vi "Input.vi"(8 "error in (no error)":errorcluster caption="错误输入（无错误）", 11 "Data In":T1) -> (0 "error out":errorcluster caption="错误输出", 3 "Data Out":T1)   [LabVIEW 2013]
uses:
  Control/Data.ctl
  Control/YV.ctl
  Control/SW.ctl
  Control/State.ctl
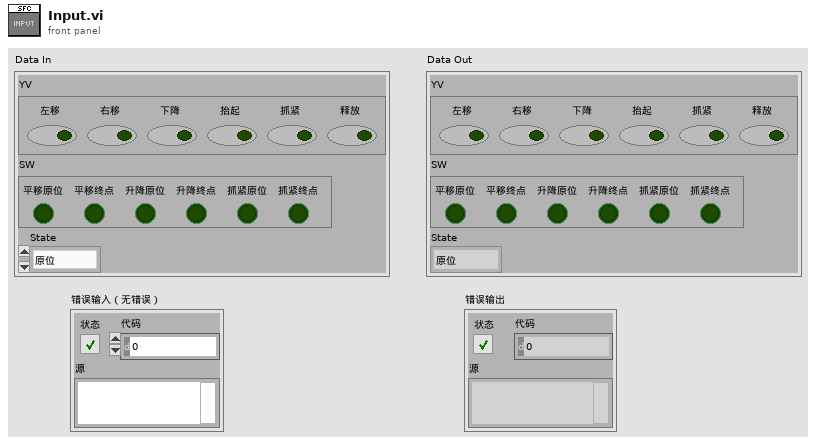
[diagram p1: front panel]
types:
  T1 = typedef "Data.ctl" = cluster{"YV":T2, "SW":T3, "State":T4}
  T2 = typedef "YV.ctl" = cluster{"左移":bool, "右移":bool, "下降":bool, "抬起":bool, "抓紧":bool, "释放":bool}
  T3 = typedef "SW.ctl" = cluster{"平移原位":bool, "平移终点":bool, "升降原位":bool, "升降终点":bool, "抓紧原位":bool, "抓紧终点":bool}
  T4 = typedef "State.ctl" = enum16{"原位", "A侧下降", "夹紧工件", "A侧抬起", "右移", "B侧下降", "释放工件", "B侧抬起", "左移"}
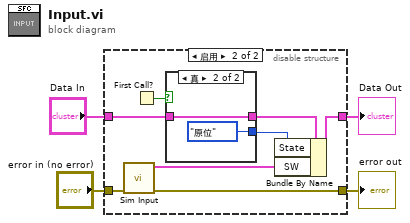
[diagram p0: block diagram]
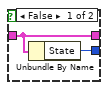
[diagram p3: hidden frame]
diagram:
  n1 = disable-structure shown="启用" {
    disable-tunnel: "Data In" -> [w6 w9]
    disable-tunnel: [w6 w14] -> w3
    disable-tunnel: "error in (no error)" -> [w5 w13]
    disable-tunnel: [w5 w12] -> w1
    frame Disabled {
    }
    frame Enabled {
      n2 = call "Sim Input.vi"("error in (no error)"=w13) -> ("error out"=w12:errorcluster, "SW Out"=w7:T3)  [unwired: 8 in]
      n3 = First Call?() -> (First Call?: T/F=w11:bool)
      n4 = case shown="真" w11 {
        tunnel: [w16 State."原位" ("State")] -> w10
        tunnel: w9 -> [w15 w17]
        tunnel: [w15 w17] -> w8
        frame False {
          n5 = Unbundle By Name(w15) -> ("State"=w16:T4)
        }
        frame True {
        }
      }
      n6 = Bundle By Name(cluster=w8, "State"=w10, "SW"=w7) -> (w14:T1)
    }
  }
  "error out" <- w1
  "Data Out" <- w3
